vi "AddToBackground.vi"(8 "error in (no error)":errorcluster, 9 "Coordinate":T1, 10 "Tilecode":u32, 11 "SnakeGame in":refnum<class "SnakeGame.lvclass">) -> (0 "error out":errorcluster, 3 "SnakeGame out":refnum<class "SnakeGame.lvclass">)   [LabVIEW 2019, in "RT_Game.lvlib" / "SnakeGame.lvclass"]
uses:
  SnakeGame.lvclass
  Game/Coordinate.ctl
  SnakeGame.lvclass/SnakeGame.ctl
  Game/Game.lvclass
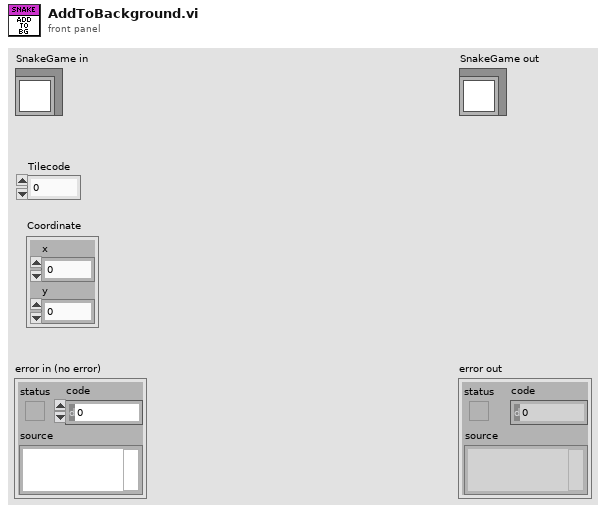
[diagram p1: front panel]
types:
  T1 = typedef "RT_Game.lvlib/Game.lvclass/Coordinate.ctl" = cluster{"x":dbl, "y":dbl}
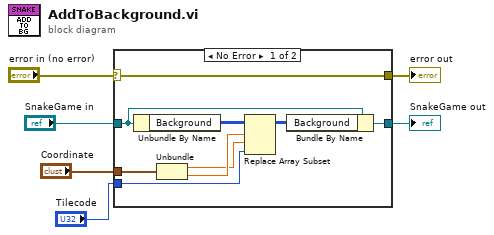
[diagram p0: block diagram]
diagram:
  n1 = case shown="No Error" "error in (no error)" {
    selector: "error in (no error)" -> [w15 w17]
    tunnel: [w15 w17] -> w5
    tunnel: [w14 w16] -> w3
    tunnel: "SnakeGame in" -> [w7 w16]
    tunnel: "Coordinate" -> [w12 _]
    tunnel: "Tilecode" -> [w11 _]
    frame No Error {
      n2 = Unbundle By Name(w7) -> ("Background"=w10:u32[][])
      n3 = Unbundle(w12) -> ("x"=w8:dbl, "y"=w9:dbl)
      n4 = Replace Array Subset(array=w10, new element=w11, index (row)=w9, index (col)=w8) -> (w13:u32[][])
      n5 = Bundle By Name(cluster=w7, "Background"=w13) -> (w14:refnum<class "SnakeGame.lvclass">)
    }
    frame Error {
    }
  }
  "error out" <- w5
  "SnakeGame out" <- w3
